vi "TagBust to Parameters.vi"(9 "Mapping":T2, 11 "parameters":T3) -> (1 "PID Parameters":T1, 3 "data table out":T3)   [LabVIEW 2015, in "PID Module 2 runtime.lvclass"]
uses:
  PID Module 2 runtime.lvclass
  <vilib>/NI/Tag Bus/table/data table.ctl
  Mapping.ctl
  PID Parameters.ctl
  <vilib>/NI/Tag Bus/table/data polymorphs/read many/read Doubles.vi
  <vilib>/NI/Tag Bus/table/data table.lvlib
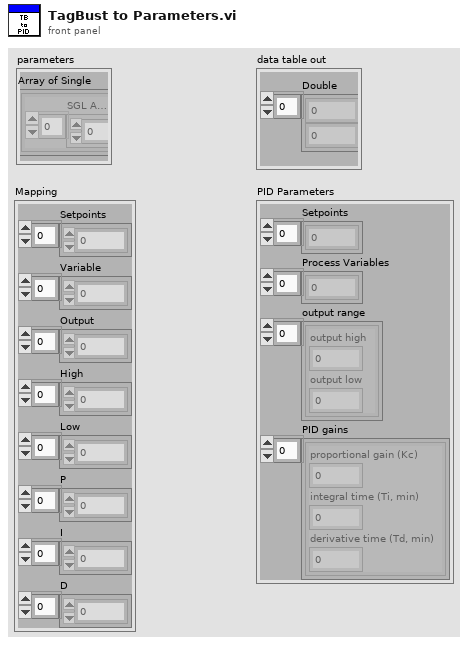
[diagram p1: front panel]
types:
  T1 = typedef "PID Module 2 runtime.lvclass/PID Parameters.ctl" = cluster{"Setpoints":dbl[], "Process Variables":dbl[], "output range":cluster{"output high":dbl, "output low":dbl}[], "PID gains":cluster{"proportional gain (Kc)":dbl, "integral time (Ti, min)":dbl, "derivative time (Td, min)":dbl}[]}
  T2 = typedef "PID Module 2 runtime.lvclass/Mapping.ctl" = cluster{"Setpoints":i32[], "Variable":i32[], "Output":i32[], "High":i32[], "Low":i32[], "P":i32[], "I":i32[], "D":i32[]}
  T3 = typedef "tag bus.lvlib/data table.lvlib/data table.ctl" = cluster{"Double":dbl[], "Single":sgl[], "I64":i64[], "I32":i32[], "I16":i16[], "I8":i8[], "U64":u64[], "U32":u32[], "U16":u16[], "U8":u8[], "Boolean":bool[], "String":string[], "Array of Double":cluster{"DBL Array":dbl[]}[], "Array of Single":cluster{"SGL Array":sgl[]}[], "Array of I64":cluster{"I64 Array":i64[]}[], "Array of I32":cluster{"I32 Array":i32[]}[], "Array of I16":cluster{"I16 Array":i16[]}[], "Array of I8":cluster{"I8 Array":i8[]}[], "Array of U64":cluster{"U64 Array":u64[]}[], "Array of U32":cluster{"U32 Array":u32[]}[], "Array of U16":cluster{"U16 Array":u16[]}[], "Array of U8":cluster{"U8 Array":u8[]}[], "Array of Boolean":cluster{"Boolean Array":bool[]}[], "Array of String":cluster{"String Array":string[]}[]}
  T4 = cluster{"proportional gain (Kc)":dbl, "integral time (Ti, min)":dbl, "derivative time (Td, min)":dbl}
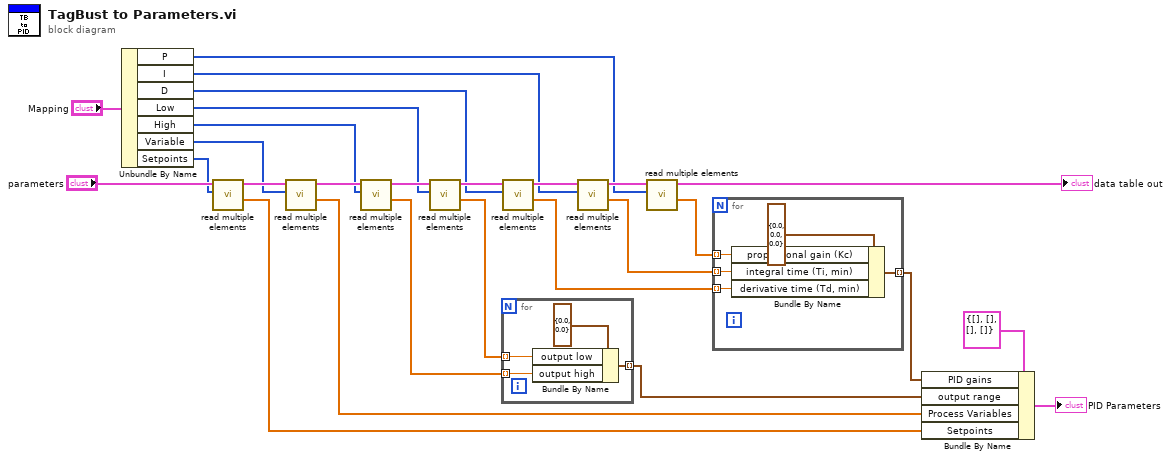
[diagram p0: block diagram]
diagram:
  n1 = Unbundle By Name("Mapping") -> ("P"=w5:i32[], "I"=w6:i32[], "D"=w7:i32[], "Low"=w15:i32[], "High"=w16:i32[], "Variable"=w19:i32[], "Setpoints"=w25:i32[])
  n2 = call-poly <vilib>:"read multiple elements.vi"("indices"=w25, "data table in"="parameters") -> ("values"=w23:dbl[], "data table out"=w21:T3)  [unwired: 8 in]
  n3 = call-poly <vilib>:"read multiple elements.vi"("indices"=w19, "data table in"=w21) -> ("values"=w20:dbl[], "data table out"=w18:T3)  [unwired: 8 in]
  n4 = call-poly <vilib>:"read multiple elements.vi"("indices"=w16, "data table in"=w18) -> ("values"=w14:dbl[], "data table out"=w17:T3)  [unwired: 8 in]
  n5 = call-poly <vilib>:"read multiple elements.vi"("indices"=w15, "data table in"=w17) -> ("values"=w13:dbl[], "data table out"=w9:T3)  [unwired: 8 in]
  n6 = for {
    tunnel: w14 -> [w30] mode=indexing
    tunnel: w13 -> [w29] mode=indexing
    tunnel: [w28] -> w12 mode=indexing
    n7 = Bundle By Name(cluster=cluster{"output high":dbl, "output low":dbl} {"output high"=0.0, "output low"=0.0} ("output range"), "output low"=w29, "output high"=w30) -> (w28:cluster{"output high":dbl, "output low":dbl})
  }
  n8 = call-poly <vilib>:"read multiple elements.vi"("indices"=w7, "data table in"=w9) -> ("values"=w2:dbl[], "data table out"=w10:T3)  [unwired: 8 in]
  n9 = call-poly <vilib>:"read multiple elements.vi"("indices"=w6, "data table in"=w10) -> ("values"=w3:dbl[], "data table out"=w11:T3)  [unwired: 8 in]
  n10 = call-poly <vilib>:"read multiple elements.vi"("indices"=w5, "data table in"=w11) -> ("values"=w4:dbl[], "data table out"=→"data table out":T3)  [unwired: 8 in]
  n11 = for {
    tunnel: w4 -> [w35] mode=indexing
    tunnel: w3 -> [w34] mode=indexing
    tunnel: w2 -> [w33] mode=indexing
    tunnel: [w32] -> w1 mode=indexing
    n12 = Bundle By Name(cluster=T4 {"proportional gain (Kc)"=0.0, "integral time (Ti, min)"=0.0, "derivative time (Td, min)"=0.0} ("PID gains"), "proportional gain (Kc)"=w35, "integral time (Ti, min)"=w34, "derivative time (Td, min)"=w33) -> (w32:T4)
  }
  n13 = Bundle By Name(cluster=T1 {"Setpoints"=[], "Process Variables"=[], "output range"=[], "PID gains"=[]}, "PID gains"=w1, "output range"=w12, "Process Variables"=w20, "Setpoints"=w23) -> (→"PID Parameters":T1)
